vi "Range to Voltage Span.vi"(5 "Range And Span":T1={"Volt Range (4 : 2V)"=4, "Enable Span (False)"=FALSE, "Lower Span (-2.0000V)"=-2.0, "Upper Span (2.0000V)"=2.0, "Bias (0)"=0.0} {"Upper Span (2.0000V)" min=-99999.0 max=99999.0 step=1.0 format="%_5g"; "Lower Span (-2.0000V)" min=-99999.0 max=99999.0 step=1.0 format="%_5g"; "Volt Range (4 : 2V)" items=["20mV", "60mV", "200mV", "1V", "2V", "6V", "20V", "50V"]}, 7 "Scaling? (False)":bool, 9 "Floating Point Position (2)":i32=2) -> (6 "Lower Span":i32=-2000 min=-99999 max=99999 step=1, 8 "Upper Span":i32=2000 min=-99999 max=99999 step=1, 10 "Bias":i32)   [LabVIEW 2020, in "Yokogawa GX Series.lvlib"]
doc: "This VI gets the voltage span value from the range."
uses:
  <instrlib>/Yokogawa GX Series/Yokogawa GX Series.lvlib
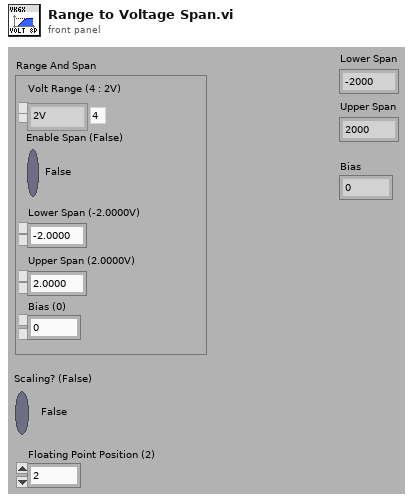
[diagram p1: front panel]
types:
  T1 = cluster{"Volt Range (4 : 2V)":i32, "Enable Span (False)":bool, "Lower Span (-2.0000V)":dbl, "Upper Span (2.0000V)":dbl, "Bias (0)":dbl}
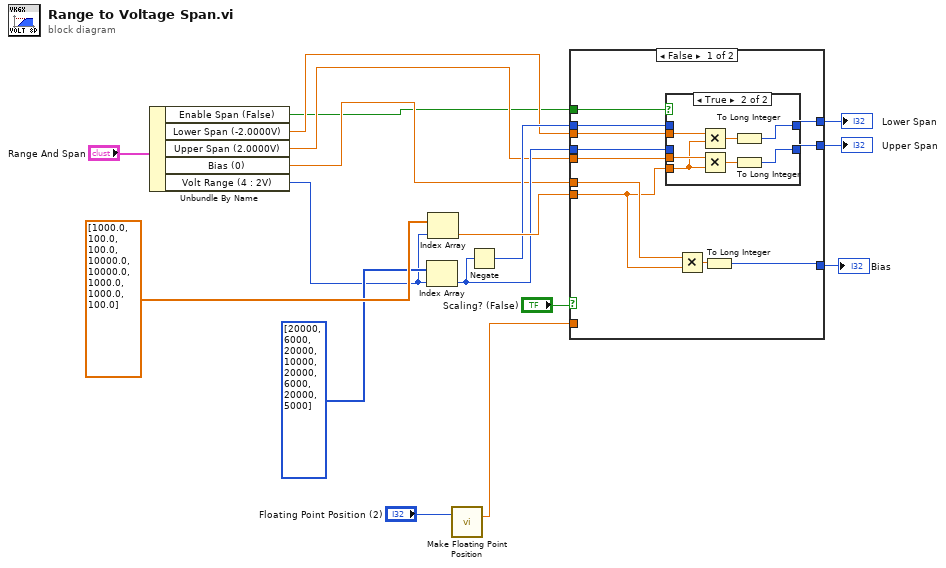
[diagram p0: block diagram]
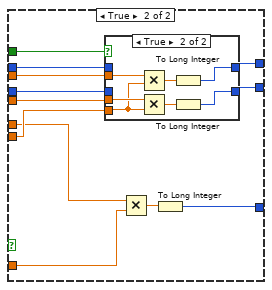
[diagram p3: hidden frame]
diagram:
  n1 = Unbundle By Name("Range And Span") -> ("Enable Span (False)"=w5:bool, "Lower Span (-2.0000V)"=w6:dbl, "Upper Span (2.0000V)"=w7:dbl, "Bias (0)"=w8:dbl, "Volt Range (4 : 2V)"=w9:i32)
  n2 = Index Array(array=i32[] [20000, 6000, 20000, 10000, 20000, 6000, 20000, 5000], index=w9) -> (element=w15:i32)
  n3 = Index Array(array=dbl[] [1000.0, 100.0, 100.0, 10000.0, 10000.0, 1000.0, 1000.0, 100.0], index=w9) -> (element=w17:dbl)
  n4 = call <instrlib>:"Make Floating Point Position.vi"("Floating Point Position (2)"="Floating Point Position (2)") -> ("Times"=w1:dbl)  [unwired: 14 in]
  n5 = Negate(x=w15) -> (-x=w16:i32)
  n6 = case shown="False" "Scaling? (False)" {
    tunnel: w17 -> [w18 w42]
    tunnel: w16 -> [w28 w49]
    tunnel: w15 -> [w27 w48]
    tunnel: [w26 w47] -> w14
    tunnel: [w25 w46] -> w13
    tunnel: [w20 w38] -> w10
    tunnel: w8 -> [w19 w39]
    tunnel: w7 -> [w24 w45]
    tunnel: w6 -> [w23 w44]
    tunnel: w5 -> [w22 w43]
    tunnel: w1 -> [_ w40]
    frame False {
      n7 = case shown="True" w22 {
        tunnel: w23 -> [_ w36]
        tunnel: w24 -> [_ w35]
        tunnel: [w30 w33] -> w26
        tunnel: [w29 w32] -> w25
        tunnel: w28 -> [w30 _]
        tunnel: w27 -> [w29 _]
        tunnel: w18 -> [_ w31]
        frame False {
        }
        frame True {
          n8 = Multiply(x=w36, y=w31) -> (x*y=w37:dbl)
          n9 = Multiply(x=w35, y=w31) -> (x*y=w34:dbl)
          n10 = To Long Integer(number=w37) -> (32bit integer=w33:i32)
          n11 = To Long Integer(number=w34) -> (32bit integer=w32:i32)
        }
      }
      n12 = Multiply(x=w19, y=w18) -> (x*y=w21:dbl)
      n13 = To Long Integer(number=w21) -> (32bit integer=w20:i32)
    }
    frame True {
      n14 = case shown="True" w43 {
        tunnel: w44 -> [_ w57]
        tunnel: w45 -> [_ w56]
        tunnel: [w51 w54] -> w47
        tunnel: [w50 w53] -> w46
        tunnel: w49 -> [w51 _]
        tunnel: w48 -> [w50 _]
        tunnel: w42 -> [_ w52]
        frame False {
        }
        frame True {
          n15 = Multiply(x=w57, y=w52) -> (x*y=w58:dbl)
          n16 = Multiply(x=w56, y=w52) -> (x*y=w55:dbl)
          n17 = To Long Integer(number=w58) -> (32bit integer=w54:i32)
          n18 = To Long Integer(number=w55) -> (32bit integer=w53:i32)
        }
      }
      n19 = Multiply(x=w39, y=w40) -> (x*y=w41:dbl)
      n20 = To Long Integer(number=w41) -> (32bit integer=w38:i32)
    }
  }
  "Lower Span" <- w14
  "Upper Span" <- w13
  "Bias" <- w10
